vi "SetpBlock.vi"(6 "PartitionList":T1(array[cluster])=[{"Check"=FALSE, "No"="001", "Frame"=2, "FrameNo"="1024Frame", "Block"=2}, {"Check"=FALSE, "No"="002", "Frame"=2, "FrameNo"="1024Frame", "Block"=2}, {"Check"=FALSE, "No"="003", "Frame"=2, "FrameNo"="1024Frame", "Block"=2}, {"Check"=FALSE, "No"="004", "Frame"=2, "FrameNo"="1024Frame", "Block"=2}, {"Check"=FALSE, "No"="005", "Frame"=2, "FrameNo"="1024Frame", "Block"=2}, {"Check"=FALSE, "No"="006", "Frame"=2, "FrameNo"="1024Frame", "Block"=2}, {"Check"=TRUE, "No"="007", "Frame"=2, "FrameNo"="1024Frame", "Block"=2}, {"Check"=FALSE, "No"="008", "Frame"=2, "FrameNo"="1024Frame", "Block"=2}, {"Check"=FALSE, "No"="", "Frame"=0, "FrameNo"="", "Block"=0}, {"Check"=FALSE, "No"="", "Frame"=0, "FrameNo"="", "Block"=0}, {"Check"=FALSE, "No"="", "Frame"=0, "FrameNo"="", "Block"=0}, {"Check"=FALSE, "No"="", "Frame"=0, "FrameNo"="", "Block"=0}, {"Check"=FALSE, "No"="", "Frame"=0, "FrameNo"="", "Block"=0}, {"Check"=FALSE, "No"="", "Frame"=0, "FrameNo"="", "Block"=0}, {"Check"=FALSE, "No"="", "Frame"=0, "FrameNo"="", "Block"=0}, {"Check"=FALSE, "No"="", "Frame"=0, "FrameNo"="", "Block"=0}, {"Check"=FALSE, "No"="", "Frame"=0, "FrameNo"="", "Block"=0}, {"Check"=FALSE, "No"="", "Frame"=0, "FrameNo"="", "Block"=0}, {"Check"=FALSE, "No"="", "Frame"=0, "FrameNo"="", "Block"=0}, {"Check"=FALSE, "No"="", "Frame"=0, "FrameNo"="", "Block"=0}, {"Check"=FALSE, "No"="", "Frame"=0, "FrameNo"="", "Block"=0}, {"Check"=FALSE, "No"="", "Frame"=0, "FrameNo"="", "Block"=0}, {"Check"=FALSE, "No"="", "Frame"=0, "FrameNo"="", "Block"=0}, {"Check"=FALSE, "No"="", "Frame"=0, "FrameNo"="", "Block"=0}, {"Check"=FALSE, "No"="", "Frame"=0, "FrameNo"="", "Block"=0}, {"Check"=FALSE, "No"="", "Frame"=0, "FrameNo"="", "Block"=0}, {"Check"=FALSE, "No"="", "Frame"=0, "FrameNo"="", "Block"=0}, {"Check"=FALSE, "No"="", "Frame"=0, "FrameNo"="", "Block"=0}, {"Check"=FALSE, "No"="", "Frame"=0, "FrameNo"="", "Block"=0}, {"Check"=FALSE, "No"="", "Frame"=0, "FrameNo"="", "Block"=0}, {"Check"=FALSE, "No"="", "Frame"=0, "FrameNo"="", "Block"=0}, {"Check"=FALSE, "No"="", "Frame"=0, "FrameNo"="", "Block"=0}, {"Check"=FALSE, "No"="", "Frame"=0, "FrameNo"="", "Block"=0}, {"Check"=FALSE, "No"="", "Frame"=0, "FrameNo"="", "Block"=0}, {"Check"=FALSE, "No"="", "Frame"=0, "FrameNo"="", "Block"=0}, {"Check"=FALSE, "No"="", "Frame"=0, "FrameNo"="", "Block"=0}, {"Check"=FALSE, "No"="", "Frame"=0, "FrameNo"="", "Block"=0}, {"Check"=FALSE, "No"="", "Frame"=0, "FrameNo"="", "Block"=0}, {"Check"=FALSE, "No"="", "Frame"=0, "FrameNo"="", "Block"=0}, {"Check"=FALSE, "No"="", "Frame"=0, "FrameNo"="", "Block"=0}, {"Check"=FALSE, "No"="", "Frame"=0, "FrameNo"="", "Block"=0}, {"Check"=FALSE, "No"="", "Frame"=0, "FrameNo"="", "Block"=0}, {"Check"=FALSE, "No"="", "Frame"=0, "FrameNo"="", "Block"=0}, {"Check"=FALSE, "No"="", "Frame"=0, "FrameNo"="", "Block"=0}, {"Check"=FALSE, "No"="", "Frame"=0, "FrameNo"="", "Block"=0}, {"Check"=FALSE, "No"="", "Frame"=0, "FrameNo"="", "Block"=0}, {"Check"=FALSE, "No"="", "Frame"=0, "FrameNo"="", "Block"=0}, {"Check"=FALSE, "No"="", "Frame"=0, "FrameNo"="", "Block"=0}, {"Check"=FALSE, "No"="", "Frame"=0, "FrameNo"="", "Block"=0}, {"Check"=FALSE, "No"="", "Frame"=0, "FrameNo"="", "Block"=0}, {"Check"=FALSE, "No"="", "Frame"=0, "FrameNo"="", "Block"=0}, {"Check"=FALSE, "No"="", "Frame"=0, "FrameNo"="", "Block"=0}, {"Check"=FALSE, "No"="", "Frame"=0, "FrameNo"="", "Block"=0}, {"Check"=FALSE, "No"="", "Frame"=0, "FrameNo"="", "Block"=0}, {"Check"=FALSE, "No"="", "Frame"=0, "FrameNo"="", "Block"=0}, {"Check"=FALSE, "No"="", "Frame"=0, "FrameNo"="", "Block"=0}, {"Check"=FALSE, "No"="", "Frame"=0, "FrameNo"="", "Block"=0}, {"Check"=FALSE, "No"="", "Frame"=0, "FrameNo"="", "Block"=0}, {"Check"=FALSE, "No"="", "Frame"=0, "FrameNo"="", "Block"=0}, {"Check"=FALSE, "No"="", "Frame"=0, "FrameNo"="", "Block"=0}, {"Check"=FALSE, "No"="", "Frame"=0, "FrameNo"="", "Block"=0}, {"Check"=FALSE, "No"="", "Frame"=0, "FrameNo"="", "Block"=0}, {"Check"=FALSE, "No"="", "Frame"=0, "FrameNo"="", "Block"=0}, {"Check"=FALSE, "No"="", "Frame"=0, "FrameNo"="", "Block"=0}], 7 "Blocks":u32[](array[numeric])=[2, 2, 2, 2, 2, 2, 2, 2, 0, 0, 0, 0, 0, 0, 0, 0, 0, 0, 0, 0, 0, 0, 0, 0, 0, 0, 0, 0, 0, 0, 0, 0, 0, 0, 0, 0, 0, 0, 0, 0, 0, 0, 0, 0, 0, 0, 0, 0, 0, 0, 0, 0, 0, 0, 0, 0, 0, 0, 0, 0, 0, 0, 0, 0], 8 "PBlock":u32=16, 9 "PCount":u32=8, 10 "NewPartitionNo":u32=8, 11 "NowPartitionNo":u32=8) -> (2 "Block":i32[](array[numeric])=[2, 2, 2, 2, 2, 2, 2, 2])   [LabVIEW 2015]
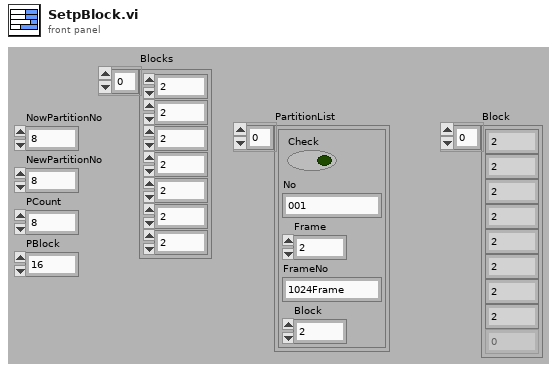
[diagram p1: front panel]
types:
  T1 = cluster{"Check":bool, "No":string, "Frame":u32, "FrameNo":string, "Block":u32}[]
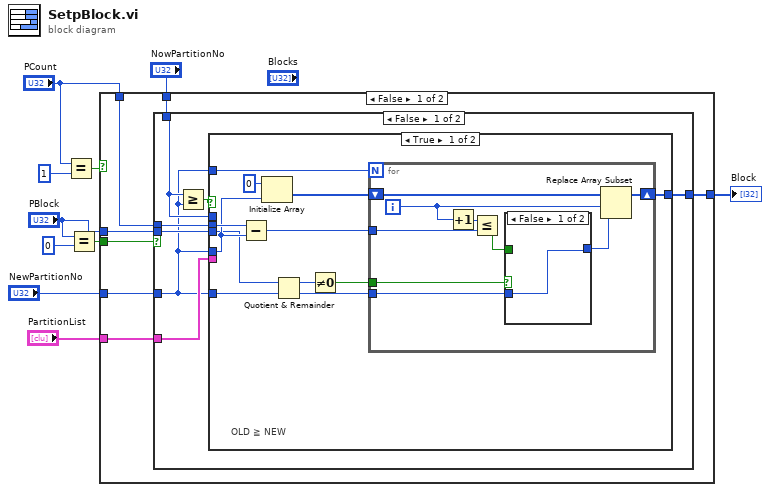
[diagram p0: block diagram]
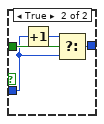
[diagram p2: hidden frame]
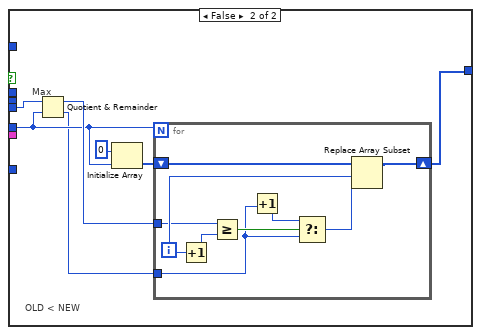
[diagram p3: hidden frame]
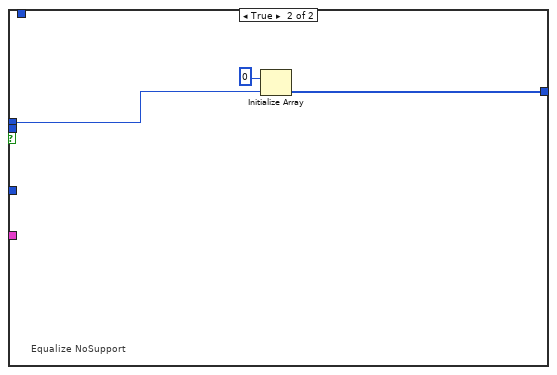
[diagram p4: hidden frame]
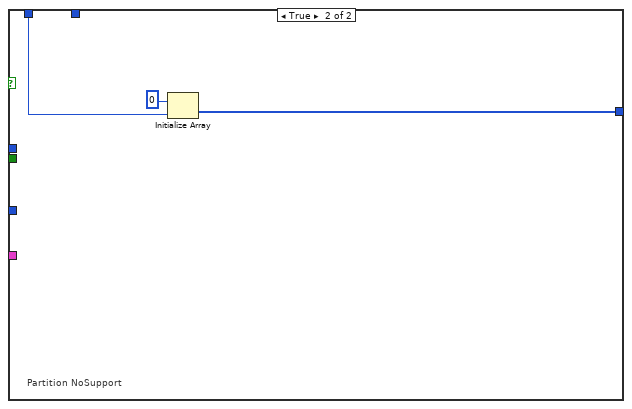
[diagram p5: hidden frame]
diagram:
  n1 = Equal?(x="PCount", y=u16 1) -> (x = y?=w5:bool)
  n2 = Equal?(x="PBlock", y=u16 0) -> (x = y?=w4:bool)
  n3 = case shown="False" w5 {
    tunnel: [w17 w70] -> w10
    tunnel: "PCount" -> [w14 w72]
    tunnel: "NewPartitionNo" -> [w16 _]
    tunnel: w4 -> [w15 _]
    tunnel: "PartitionList" -> [w13 _]
    tunnel: "NowPartitionNo" -> [w12 _]
    tunnel: "PBlock" -> [w11 _]
    frame False {
      n4 = case shown="False" w15 {
        tunnel: [w24 w68] -> w17
        tunnel: w16 -> [w18 _]
        tunnel: w14 -> [w21 w67]
        tunnel: w13 -> [w23 _]
        tunnel: w12 -> [w20 _]
        tunnel: w11 -> [w19 _]
        frame False {
          n5 = Greater Or Equal?(x=w20, y=w18) -> (x >= y?=w22:bool)
          n6 = case shown="True" w22 {
            tunnel: [w36 w52] -> w24
            tunnel: w23 -> [_ _]
            tunnel: w21 -> [w33 _]
            tunnel: w18 -> [w32 w55]
            tunnel: w18 -> [w30 _]
            tunnel: w20 -> [_ _]
            tunnel: w19 -> [w29 w51]
            tunnel: w18 -> [w28 _]
            frame True {
              # "OLD ≧ NEW"
              n7 = Subtract(x=w33, y=w32) -> (x-y=w31:u32)
              n8 = Initialize Array(0, w32) -> (w34:i32[])
              n9 = Quotient & Remainder(x=w29, y=w28) -> (x-y*floor(x/y)=w26:u32, floor(x/y)=w27:u32)
              n10 = Not Equal To 0?(x=w26) -> (x != 0?=w25:bool)
              n11 = for {
                N: w30 -> [_]
                shift-right: [w44] -> w36
                shift-left: w34 -> [w45]
                tunnel: w31 -> [w41]
                tunnel: w27 -> [w38]
                tunnel: w25 -> [w37]
                i -> [w43]
                n12 = Increment(x=w43) -> (x+1=w42:i32)
                n13 = Less Or Equal?(x=w42, y=w41) -> (x <= y?=w40:bool)
                n14 = case shown="False" w37 {
                  tunnel: w40 -> [_ w50]
                  tunnel: [w46 w49] -> w39
                  tunnel: w38 -> [w46 w47]
                  frame False {
                  }
                  frame True {
                    n15 = Increment(x=w47) -> (x+1=w48:u32)
                    n16 = Select(t=w48, s=w50, f=w47) -> (s? t:f=w49:u32)
                  }
                }
                n17 = Replace Array Subset(array=w45, new element=w39, index=w43) -> (w44:i32[])
              }
            }
            frame False {
              # "OLD < NEW"
              # "Max"
              n18 = Quotient & Remainder(x=w51, y=w55) -> (x-y*floor(x/y)=w57:u32, floor(x/y)=w53:u32)
              n19 = Initialize Array(0, w55) -> (w54:i32[])
              n20 = for {
                N: w55 -> [_]
                tunnel: w57 -> [w64]
                shift-right: [w58] -> w52
                shift-left: w54 -> [w66]
                tunnel: w53 -> [w61]
                i -> [w65]
                n21 = Increment(x=w65) -> (x+1=w63:i32)
                n22 = Greater Or Equal?(x=w64, y=w63) -> (x >= y?=w62:bool)
                n23 = Increment(x=w61) -> (x+1=w60:u32)
                n24 = Select(t=w60, s=w62, f=w61) -> (s? t:f=w59:u32)
                n25 = Replace Array Subset(array=w66, new element=w59, index=w65) -> (w58:i32[])
              }
            }
          }
        }
        frame True {
          # "Equalize NoSupport"
          n26 = Initialize Array(0, w67) -> (w68:i32[])
        }
      }
    }
    frame True {
      # "Partition NoSupport"
      n27 = Initialize Array(0, w72) -> (w70:i32[])
    }
  }
  "Block" <- w10
